vi "up2PWM.vi"() -> ()   [LabVIEW 2021]
panel:
  out "PWM":dbl
  in  "up":dbl
  out "error out":errorcluster
  in  "error in (no error)":errorcluster
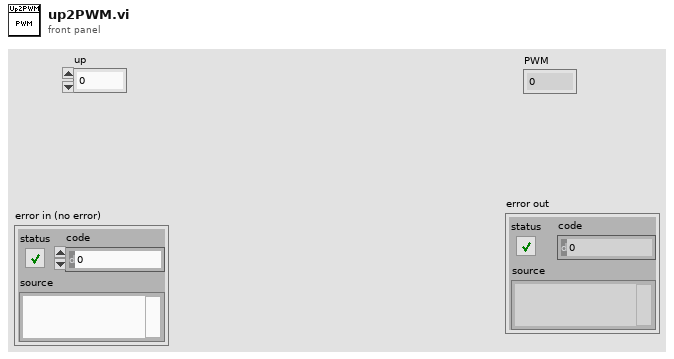
[diagram p1: front panel]
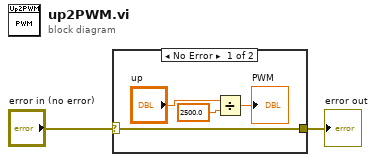
[diagram p0: block diagram]
diagram:
  n1 = case shown="No Error" "error in (no error)" {
    selector: "error in (no error)" -> [w6 w7]
    tunnel: [w6 w7] -> w1
    frame No Error {
      n2 = Divide(x="up", y=2500.0) -> (x/y=→"PWM":dbl)
    }
    frame Error {
    }
  }
  "error out" <- w1
